vi "Fill.vi"(8 "error in (no error)":errorcluster, 10 "Color":refnum<k24>, 11 "Canvas in":refnum<class "Drawer .Net.lvclass">) -> (0 "error out":errorcluster, 3 "Canvas out":refnum<class "Drawer .Net.lvclass">)   [LabVIEW 2020, in "Glyph .NET.lvlib" / "Drawer .Net.lvclass"]
uses:
  Drawer .Net.lvclass
  System.Drawing
  Drawer .Net.lvclass/Drawer .Net.ctl
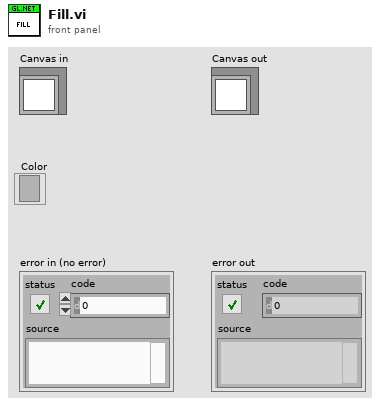
[diagram p1: front panel]
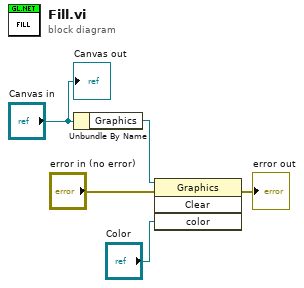
[diagram p0: block diagram]
diagram:
  n1 = Unbundle By Name("Canvas in") -> ("Graphics"=w1:refnum<k24>)
  n2 = invoke class="Graphics" method="Clear"(reference=w1, error in="error in (no error)", "color"="Color") -> (error out=→"error out":errorcluster)  [unwired: 1 in, 3 out]
  "Canvas out" <- "Canvas in"
